vi "Untitled 2.vi"() -> ()   [LabVIEW 2012]
panel:
  out "?":bool[](array[boolean])=[TRUE, TRUE, TRUE, TRUE, TRUE, TRUE, TRUE, TRUE, FALSE, FALSE, FALSE, FALSE, FALSE, FALSE, FALSE, FALSE, FALSE, FALSE, FALSE, FALSE, FALSE, FALSE, FALSE, FALSE, FALSE, FALSE, FALSE, FALSE, FALSE, FALSE, FALSE, FALSE, FALSE, FALSE, FALSE, FALSE, FALSE, FALSE, FALSE, FALSE, FALSE, FALSE, FALSE, FALSE, FALSE, FALSE, FALSE, FALSE, FALSE, FALSE, FALSE, FALSE, FALSE, FALSE, FALSE, FALSE, FALSE, FALSE, FALSE, FALSE, FALSE, FALSE, FALSE, FALSE]
  out "REG 97":u32=255
  in  "DAC_TH2":u32
  in  "DAC_TH5":u32=255
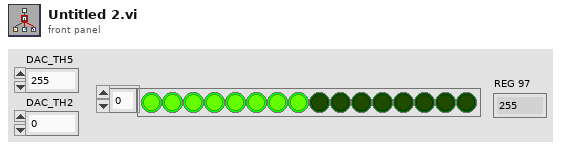
[diagram p1: front panel]
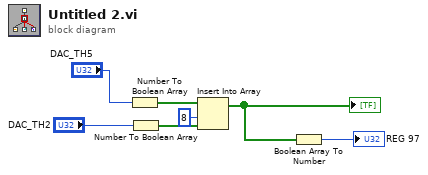
[diagram p0: block diagram]
diagram:
  n1 = Number To Boolean Array(number="DAC_TH5") -> (Boolean array=w5:bool[])
  n2 = Number To Boolean Array(number="DAC_TH2") -> (Boolean array=w4:bool[])
  n3 = Insert Into Array(array=w5, index=8, new element=w4) -> (w3:bool[])
  "?" <- w3
  n4 = Boolean Array To Number(Boolean array=w3) -> (number=→"REG 97":u32)
